vi "tsdb_unload_can_db_win32.vi"(8 "错误输入（无错误）":errorcluster, 11 "out AId":u32) -> (0 "错误输出":errorcluster, 3 "tsdb_unload_can_db":i32)   [LabVIEW 2016]
uses:
  TSMaster.dll
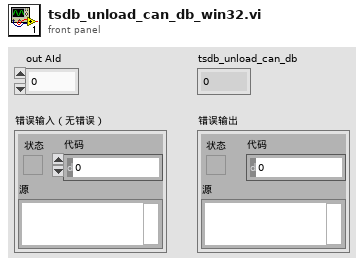
[diagram p1: front panel]
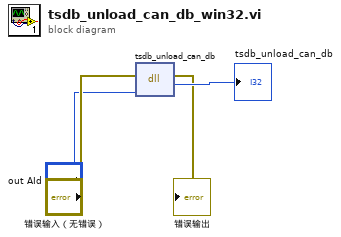
[diagram p0: block diagram]
diagram:
  n1 = dll-call lib="C:/Users/Eric/Desktop/LabVIEW/TSMasterAPI/Win32/TSMaster_LV2010_Release/TSMaster.dll" fn="tsdb_unload_can_db"(error in="错误输入（无错误）", "AId"="out AId") -> (error out=→"错误输出":errorcluster, "tsdb_unload_can_db"=→"tsdb_unload_can_db":i32)  [unwired: 3 in, 1 out]
